vi "Nanodac_lectura.vi"(0 "Modbus Master in":refnum<class "Modbus Master.lvclass">, 5 "error in (no error)":errorcluster) -> (14 "Modbus Master out":refnum<class "Modbus Master.lvclass">, 16 "O2, CO, LEL":dbl[](array[numeric]), 17 "O2, CO, LEL":bool[](array[boolean]), 19 "error out":errorcluster)   [LabVIEW 2022 SP3, in "CC_Library.lvlib"]
uses:
  CC_Library.lvlib
  <vilib>/Modbus/master/Modbus Master.lvclass
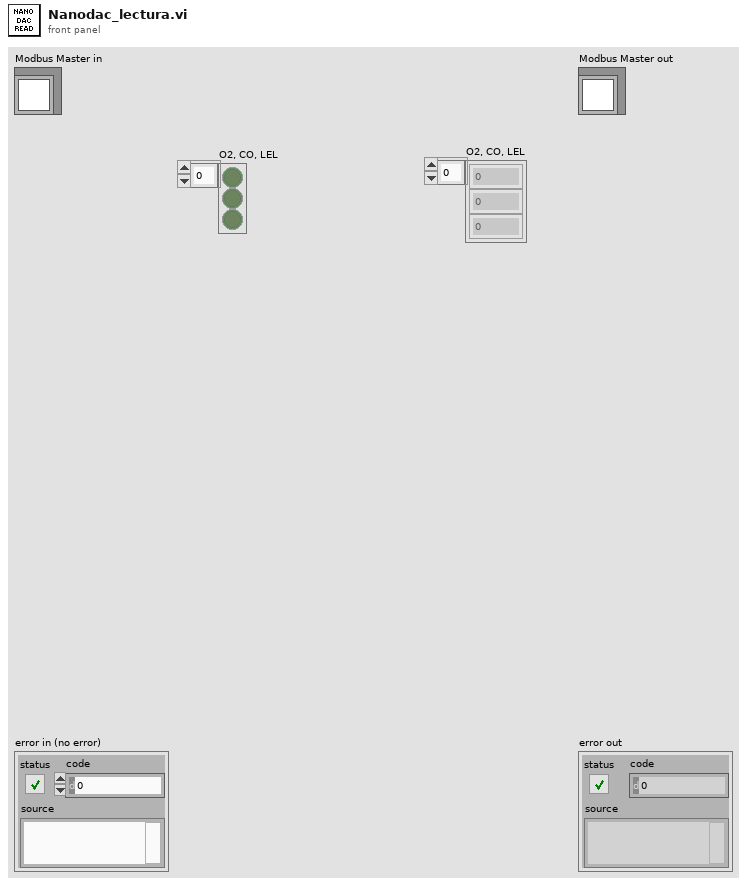
[diagram p1: front panel]
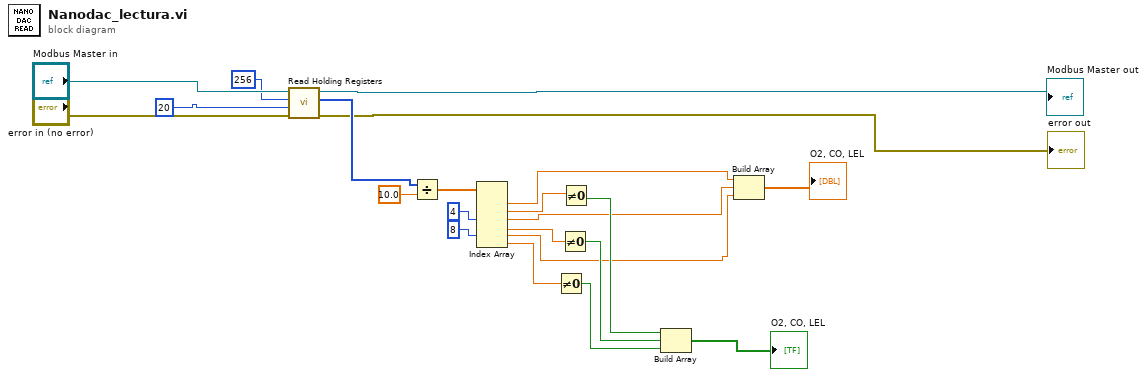
[diagram p0: block diagram]
diagram:
  n1 = call-dynamic "Read Holding Registers.vi"("error in (no error)"="error in (no error)", "number of holding registers"=u16 20, "starting address"=u16 256 ("address"), "Modbus master in"="Modbus Master in") -> ("error out"=→"error out":errorcluster, "register values"=w21:u16[], "Modbus master out"=→"Modbus Master out":refnum<class "Modbus Master.lvclass">)  [unwired: 5 in]
  n2 = Divide(x=w21, y=10.0) -> (x/y=w10:dbl[])
  n3 = Index Array(array=w10, index #3=4 ("index"), index #5=8 ("index")) -> (element #1=w4:dbl, element #2=w15:dbl, element #3=w3:dbl, element #4=w13:dbl, element #5=w2:dbl, element #6=w14:dbl)  [unwired: 4 in]
  n4 = Not Equal To 0?(x=w14) -> (x != 0?=w6:bool)
  n5 = Not Equal To 0?(x=w13) -> (x != 0?=w7:bool)
  n6 = Not Equal To 0?(x=w15) -> (x != 0?=w8:bool)
  n7 = Build Array(w8, w7, w6) -> (→"O2, CO, LEL":bool[])
  n8 = Build Array(w4, w3, w2) -> (→"O2, CO, LEL":dbl[])
